vi "判断连零.vi"(1 "原消息代码":dbl[](array[numeric])) -> (0 "布尔":bool)   [LabVIEW 2013]
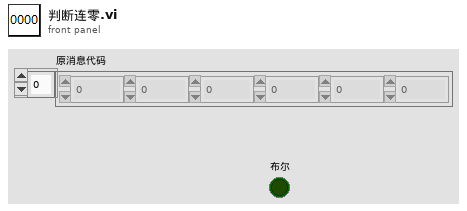
[diagram p1: front panel]
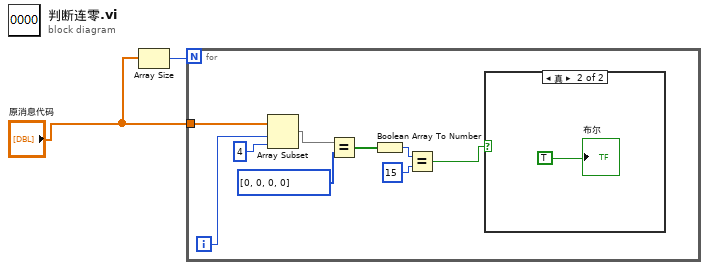
[diagram p0: block diagram]
diagram:
  n1 = Array Size(array="原消息代码") -> (size(s)=w2:i32)
  n2 = for {
    N: w2 -> [_]
    tunnel: "原消息代码" -> [w11]
    i -> [w10]
    n3 = Array Subset(array=w11, index=w10, length=4) -> (w8:dbl[])
    n4 = Equal?(x=w8, y=i32[] [0, 0, 0, 0]) -> (x = y?=w6:bool[])
    n5 = Boolean Array To Number(Boolean array=w6) -> (number=w5:u32)
    n6 = Equal?(x=w5, y=15) -> (x = y?=w3:bool)
    n7 = case shown="真" w3 {
      frame False {
      }
      frame True {
        "布尔" <- TRUE
      }
    }
  }
